vi "4.vi"   [LabVIEW 2017]
uses:
  <vilib>/measure/NI_MABase.lvlib
types:
  T1 = enum16{"open", "replace", "create", "open or create", "replace or create", "replace or create with confirmation"}
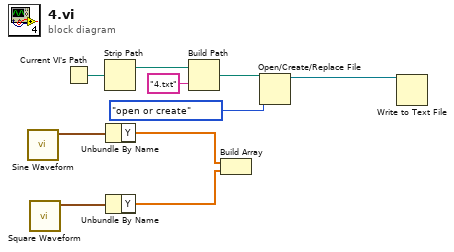
[diagram p0: block diagram]
diagram:
  n1 = call <vilib>:"Sine Waveform.vi"() -> ("signal out"=w11:waveform(dbl))  [unwired: 10 in, 1 out]
  n2 = call <vilib>:"Square Waveform.vi"() -> ("signal out"=w10:waveform(dbl))  [unwired: 10 in, 1 out]
  n3 = Current VI's Path() -> (path=w6:path)
  n4 = Strip Path(path=w6) -> (stripped path=w5:path)  [unwired: 1 out]
  n5 = Unbundle By Name(w11) -> ("Y"=w9:dbl[])
  n6 = Unbundle By Name(w10) -> ("Y"=w8:dbl[])
  n7 = Build Path(base path=w5, name or relative path="4.txt" ("名称或相对路径")) -> (appended path=w3:path)
  n8 = Build Array(w9, w8) -> (w7:dbl[][])
  n9 = Open/Create/Replace File(file path (use dialog)=w3, operation (0:open)=T1."open or create" ("操作(0:open)")) -> (refnum out=w1:refnum<file>)  [unwired: 4 in, 2 out]
  n10 = Write to Text File(file (use dialog)=w1) -> ()  [unwired: 3 in, 3 out]
